vi "Limit_I16.vi"(8 "Limit":i16, 9 "I16":i16) -> (3 "out":i16)   [LabVIEW 2018]
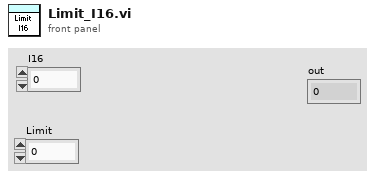
[diagram p1: front panel]
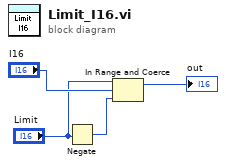
[diagram p0: block diagram]
diagram:
  n1 = Negate(x="Limit") -> (-x=w3:i16)
  n2 = In Range and Coerce(upper limit="Limit", x="I16", lower limit=w3) -> (coerced(x)=→"out":i16)  [unwired: 1 out]
